vi "Build Tx Cluster.vi"(8 "error in":errorcluster, 11 "custom device ref in":T5=18446744073709551615 format="%.0x") -> (0 "error out":errorcluster, 2 "Tx cluster out":T1 {"channel settings"."Frame Array"."Data" format="%.0x"; "channel settings"."Frame Array"."HeaderInfo"."NetSelect" items=["FDX_TX_FRAME_DLY_A"=0, "FDX_TX_FRAME_DLY_B"=1, "FDX_TX_FRAME_BOTH "=3, "FDX_TX_FRAME_ONLY_A"=4, "FDX_TX_FRAME_ONLY_B "=5]; "channel settings"."Frame Array"."HeaderInfo"."FrameStartMode" items=["FDX_TX_FRAME_START_IFG", "FDX_TX_FRAME_START_PGWT", "FDX_TX_FRAME_START_TRG"]; "channel settings"."Frame Array"."HeaderInfo"."PhysErrorInjection" items=["FDX_TX_FRAME_ERR_OFF"=0, "FDX_TX_FRAME_ERR_CRC"=1, "FDX_TX_FRAME_ERR_ALI"=2, "FDX_TX_FRAME_ERR_PRE"=4, "FDX_TX_FRAME_ERR_PHY"=8]; "channel settings"."Frame Array"."HeaderInfo"."SequenceNumberInit" items=["FDX_TX_FRAME_SEQ_INIT_AUTO"=65535]; "channel settings"."Frame Array"."HeaderInfo"."SequenceNumberOffset" items=["FDX_TX_FRAME_SEQ_OFFS_AUTO "=65535]; "channel settings"."Frame Array"."HeaderInfo"."PayloadGenerationMode" items=["FDX_TX_FRAME_PGM_USER"=0, "FDX_TX_FRAME_PGM_IP_PART"=1, "FDX_TX_FRAME_PGM_IP_FULL"=2, "FDX_TX_FRAME_PGM_IP_PART_TT"=10, "FDX_TX_FRAME_PGM_IP_FULL_TT"=20]; "channel settings"."Frame Array"."HeaderInfo"."PayloadBufferMode" items=["FDX_TX_FRAME_PBM_STD", "FDX_TX_FRAME_PBM_MAC", "FDX_TX_FRAME_PBM_UDP"]}, 3 "custom device ref out":T5 format="%.0x")   [LabVIEW 2020, in "AIM ARINC 664 Scripting.lvlib"]
uses:
  AIM ARINC 664 Scripting.lvlib
  <vilib>/NI VeriStand/Custom Device API/Custom Device API.lvlib
  <vilib>/NI VeriStand/Custom Device API/Get Item Property (U32).vi
  Constants.vi
  <instrlib>/AIM GmbH/_AIM 664/_controls/queue_header_generic.ctl
  <instrlib>/AIM GmbH/_AIM 664/AIM664LV.lvlib
  Engine/Implementation/Tx Execution Unit/channel_settings_tx.ctl
  Engine/Implementation/Tx Execution Unit/Tx Generic Execution Unit.lvclass
  Engine/Implementation/Tx Execution Unit/hardware_channels_tx.ctl
  Engine/Implementation/Tx Execution Unit/RawFrame.ctl
  <vilib>/Utility/SystemLogging/NI_SystemLogging.lvlib
  <vilib>/NI VeriStand/Custom Device API/Custom Device Item Ref.ctl
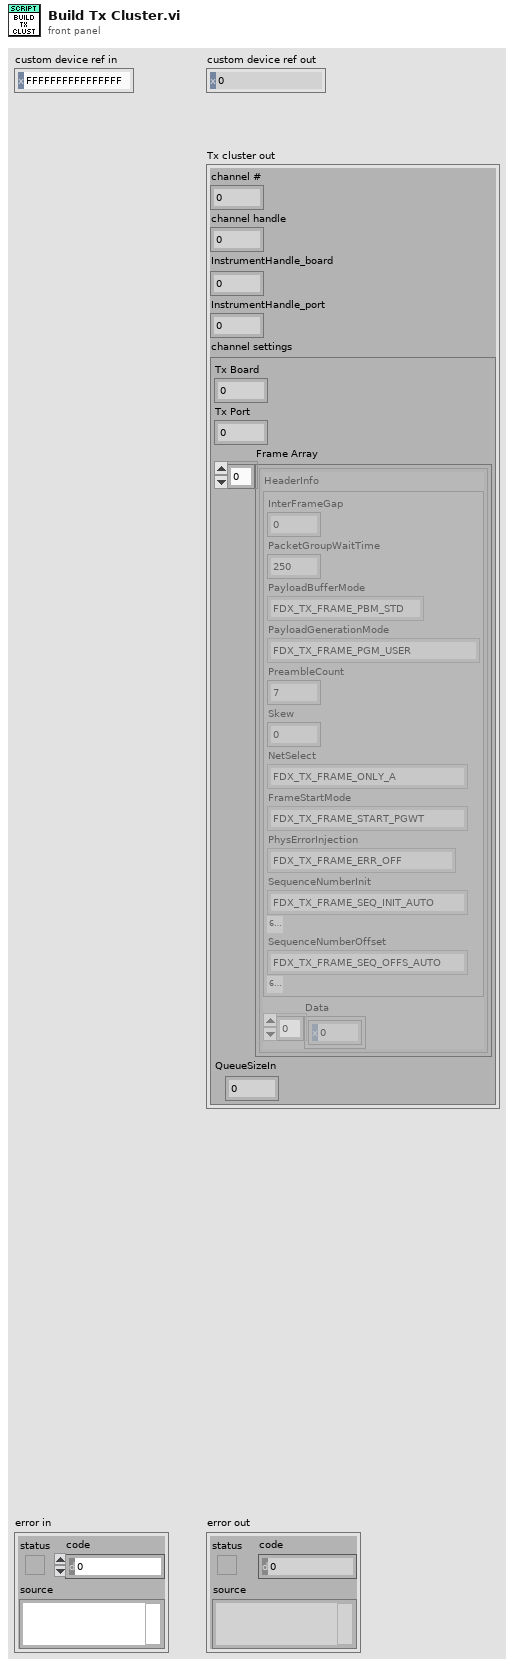
[diagram p1: front panel]
types:
  T1 = typedef "AIM ARINC 664 Engine.lvlib/Implementation.lvlib/Tx Generic Execution Unit.lvclass/hardware_channels_tx.ctl" = cluster{"channel #":u16, "channel handle":u64, "InstrumentHandle_board":u32, "InstrumentHandle_port":u32, "channel settings":T2}
  T2 = typedef "AIM ARINC 664 Engine.lvlib/Implementation.lvlib/Tx Generic Execution Unit.lvclass/channel_settings_tx.ctl" = cluster{"Tx Board":u32, "Tx Port":u32, "Frame Array":T3[], "QueueSizeIn":u32}
  T3 = typedef "AIM ARINC 664 Engine.lvlib/Implementation.lvlib/Tx Generic Execution Unit.lvclass/RawFrame.ctl" = cluster{"HeaderInfo":T4, "Data":u8[]}
  T4 = typedef "AIM664LV.lvlib/queue_header_generic.ctl" = cluster{"InterFrameGap":u32, "PacketGroupWaitTime":u32, "PayloadBufferMode":u8, "PayloadGenerationMode":u8, "PreambleCount":u8, "Skew":u32, "NetSelect":u8, "FrameStartMode":u8, "PhysErrorInjection":u32, "SequenceNumberInit":u16, "SequenceNumberOffset":u16}
  T5 = typedef "Custom Device API.lvlib/Custom Device Item Ref.ctl" = u64
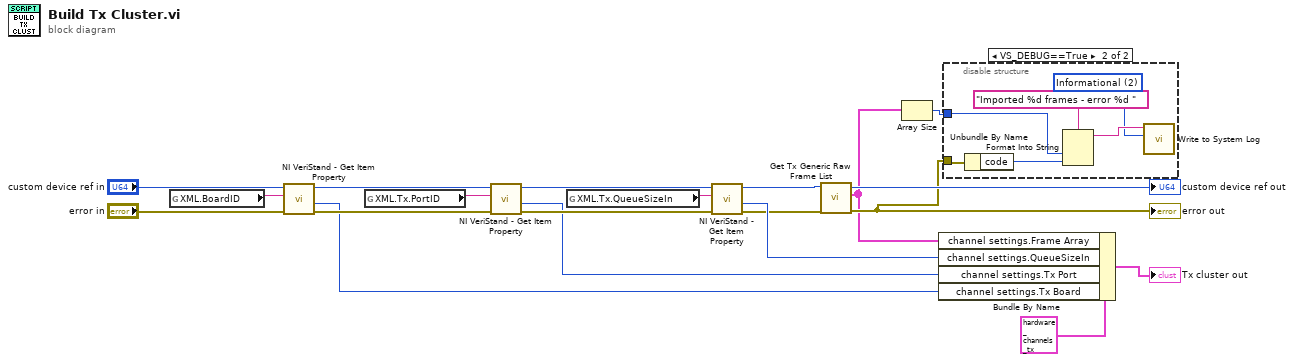
[diagram p0: block diagram]
diagram:
  n1 = global read "Constants.vi" "XML.BoardID"() -> (w14:string)
  n2 = call-poly <vilib>:"NI VeriStand - Get Item Property.vi"("error in (no error)"="error in", "Property Name"=w14, "Item Ref in"="custom device ref in") -> ("error out"=w16:errorcluster, "Value"=w10:u32, "Item Ref out"=w19:T5)  [unwired: 5 in, 1 out]
  n3 = global read "Constants.vi" "XML.Tx.PortID"() -> (w13:string)
  n4 = call-poly <vilib>:"NI VeriStand - Get Item Property.vi"("error in (no error)"=w16, "Property Name"=w13, "Item Ref in"=w19) -> ("error out"=w15:errorcluster, "Value"=w8:u32, "Item Ref out"=w18:T5)  [unwired: 5 in, 1 out]
  n5 = global read "Constants.vi" "XML.Tx.QueueSizeIn"() -> (w12:string)
  n6 = call-poly <vilib>:"NI VeriStand - Get Item Property.vi"("error in (no error)"=w15, "Property Name"=w12, "Item Ref in"=w18) -> ("error out"=w6:errorcluster, "Value"=w9:u32, "Item Ref out"=w5:T5)  [unwired: 5 in, 1 out]
  n7 = call "Get Tx Generic Raw Frame List.vi"("error in"=w6, "custom device ref in"=w5) -> ("error out"=w3:errorcluster, "Raw Frame List"=w2:T3[], "custom device ref out"=→"custom device ref out":T5)  [unwired: 6 in, 1 out]
  "error out" <- w3
  n8 = Array Size(array=w2) -> (size(s)=w1:i32)
  n9 = Bundle By Name(cluster=T1 {"channel #"=0, "channel handle"=0, "InstrumentHandle_board"=0, "InstrumentHandle_port"=0, "channel settings"={"Tx Board"=0, "Tx Port"=0, "Frame Array"=[{"HeaderInfo"={"InterFrameGap"=0, "PacketGroupWaitTime"=250, "PayloadBufferMode"=0, "PayloadGenerationMode"=0, "PreambleCount"=7, "Skew"=0, "NetSelect"=4, "FrameStartMode"=1, "PhysErrorInjection"=0, "SequenceNumberInit"=65535, "SequenceNumberOffset"=65535}, "Data"=[]}, {"HeaderInfo"={"InterFrameGap"=0, "PacketGroupWaitTime"=250, "PayloadBufferMode"=0, "PayloadGenerationMode"=0, "PreambleCount"=7, "Skew"=0, "NetSelect"=4, "FrameStartMode"=1, "PhysErrorInjection"=0, "SequenceNumberInit"=65535, "SequenceNumberOffset"=65535}, "Data"=[]}], "QueueSizeIn"=0}} ("TX Parameters"), "channel settings.Frame Array"=w2, "channel settings.QueueSizeIn"=w9, "channel settings.Tx Port"=w8, "channel settings.Tx Board"=w10) -> (→"Tx cluster out":T1)
  n10 = disable-structure shown="VS_DEBUG==True" {
    disable-tunnel: w3 -> [_ w23]
    disable-tunnel: w1 -> [_ w21]
    frame condition #0 {
    }
    frame condition #1 (active) {
      w24 = 2 items=["Error", "Warning", "Informational"] ("severity")
      n11 = Unbundle By Name(w23) -> ("code"=w22:i32)
      n12 = Format Into String(format string="Imported %d frames - error %d ", w21, w22) -> (resulting string=w25:string)  [unwired: 2 in, 1 out]
      n13 = call <vilib>:"Write to System Log.vi"("severity"=w24, "message"=w25) -> ()  [unwired: 9 in, 1 out]
    }
  }
